vi "analog Handler.vi"(0 "Variable Index":i32, 1 "Action":T2, 5 "End Tid":dbl, 7 "Value":dbl, 9 "Upd freq":T1, 11 "error in (no error)":errorcluster, 12 "Start tid / buf size":dbl, 13 "Initial Data":dbl[](array[numeric])) -> (3 "Indexes":i32[](array[numeric]), 6 "Value out":dbl, 8 "Waveform":waveform(sgl), 10 "Values":dbl[](array[numeric]), 14 "Numb var":i32, 15 "error out":errorcluster)   [LabVIEW 2011]
uses:
  Action Analog Handler.ctl
  Update frequensies.ctl
  Analog Psudo WF.ctl
panel:
  out "Time Stamp":timestamp
  # "OBS, \nBruk Value som oppdaterings frekvens \nunder reg new var."
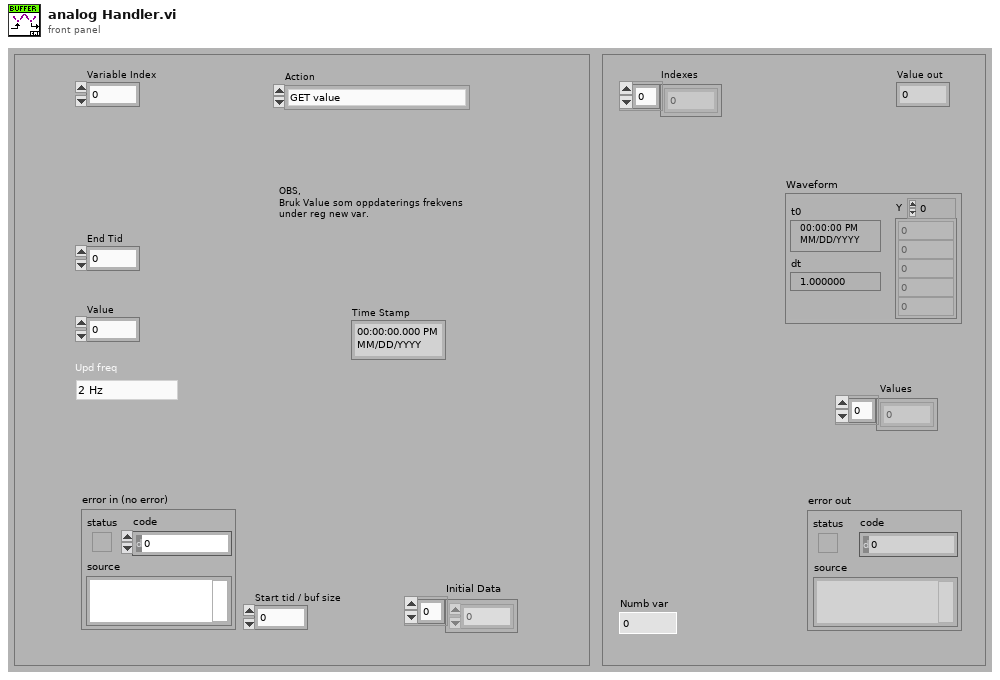
[diagram p1: front panel]
types:
  T1 = typedef "Update frequensies.ctl" = enum16{"2 Hz", "1 Hz", "0.1 Hz"}
  T2 = typedef "Action Analog Handler.ctl" = enum16{"GET value", "GET Single Frequenzy", "GET All Values", "GET Waveform", "Get Numb Var", "SET Value", "START Buffer", "REG Variable", "BUF size(total antal sekund)", "PULS", "Get a Value at time", "Set initial waveform"}
  T3 = typedef "Analog Psudo WF.ctl" = cluster{"\ndata":sgl[], "Index":i32, "Upd freq":T1, "Last index time":dbl, "Rounded":bool}
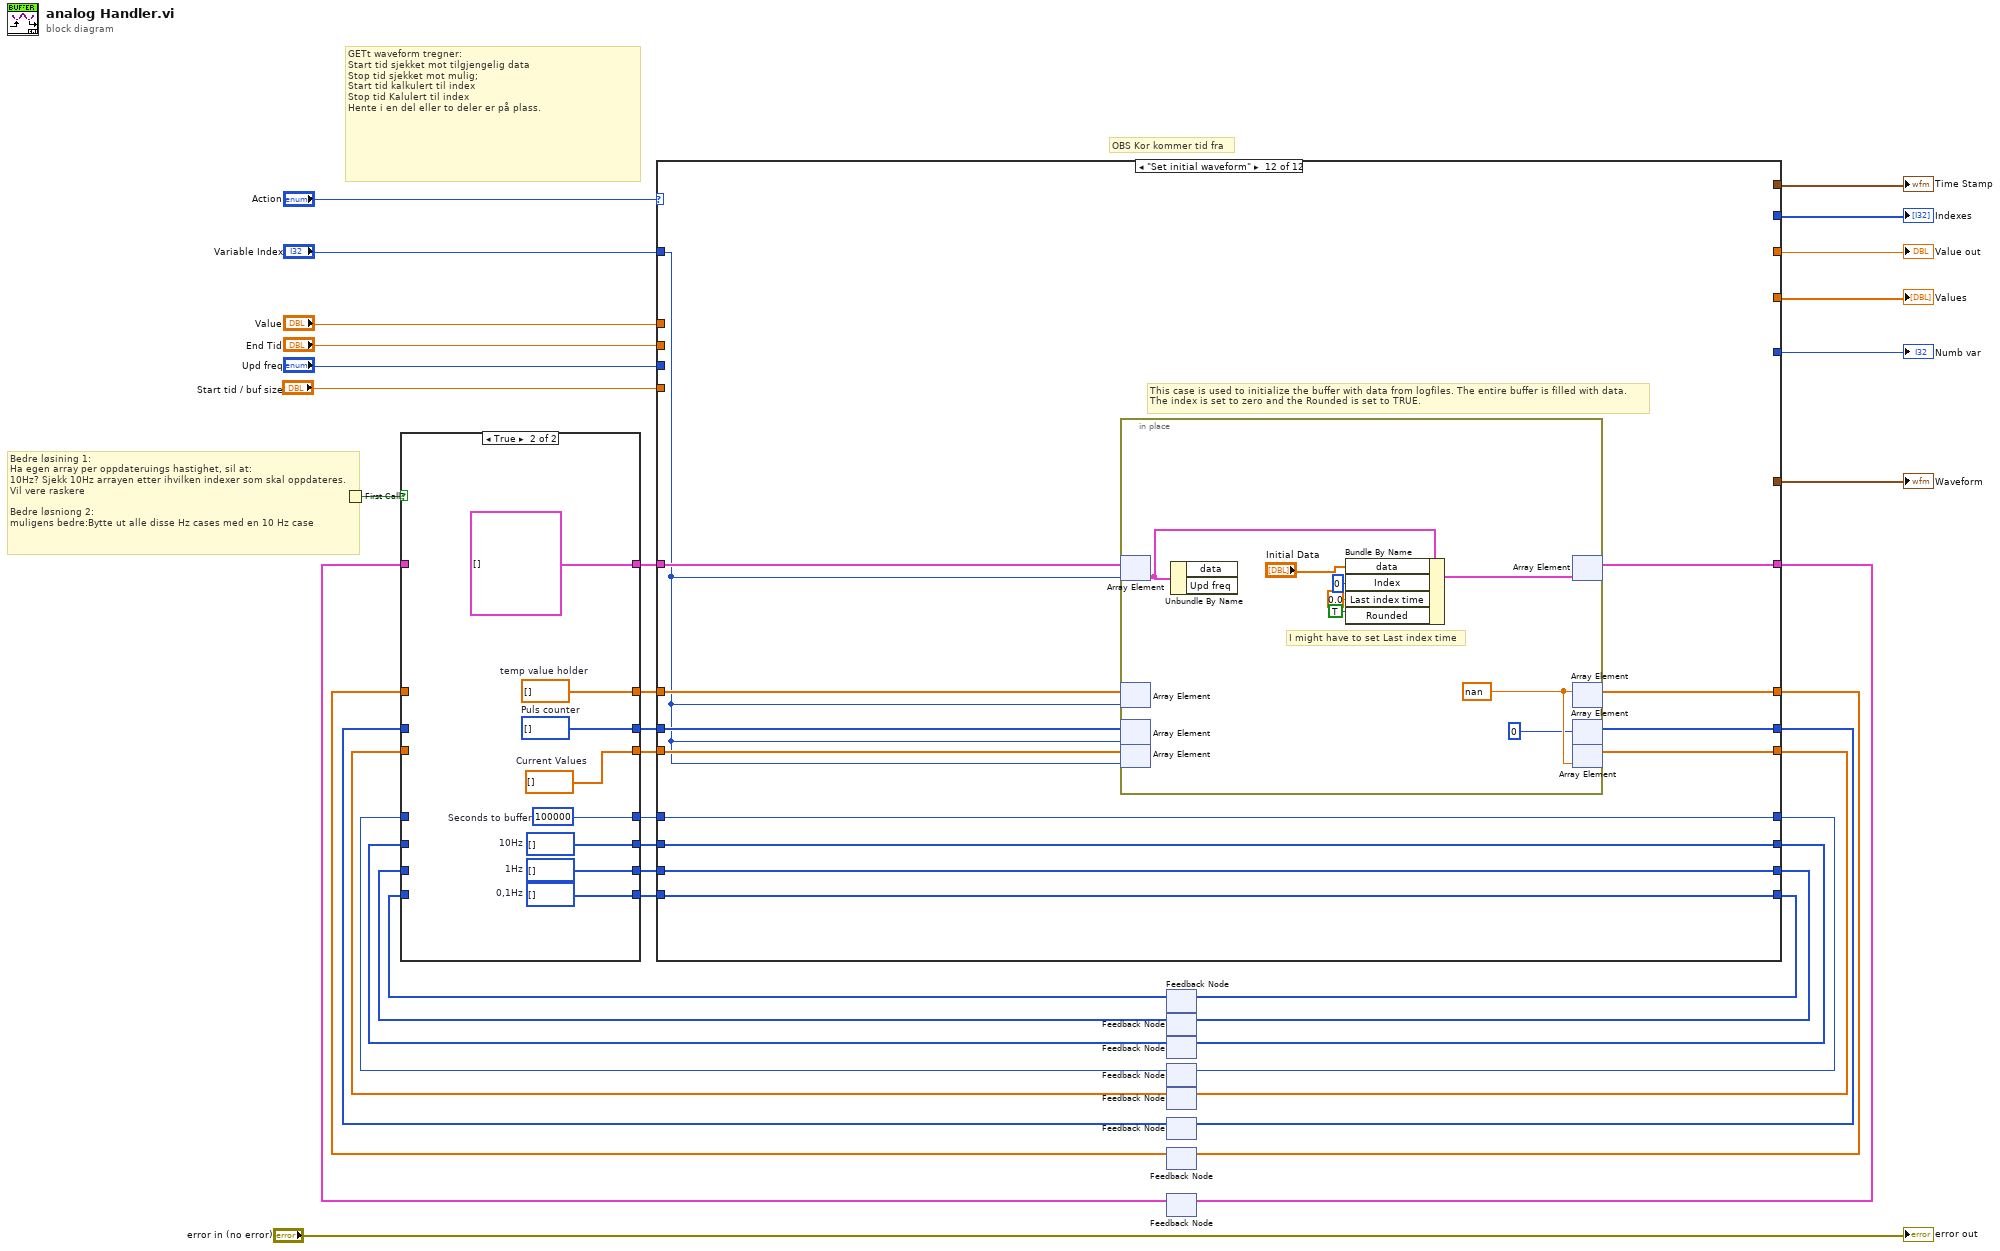
[diagram p0: block diagram]
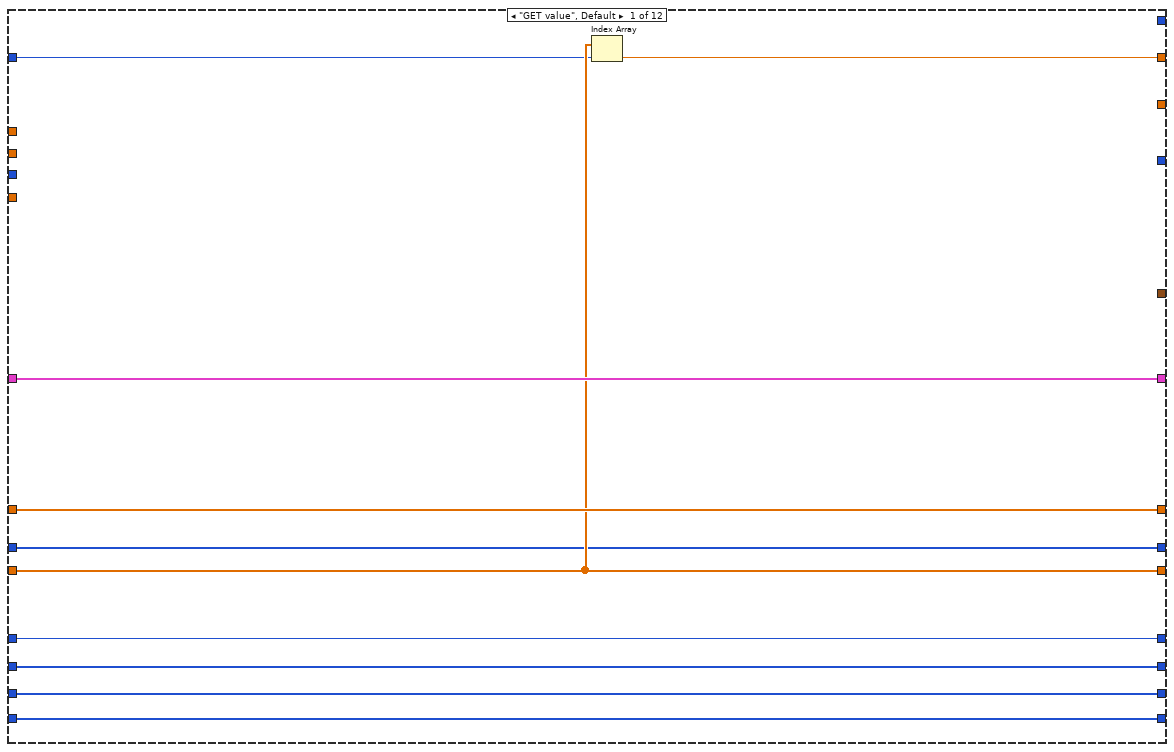
[diagram p3: hidden frame]
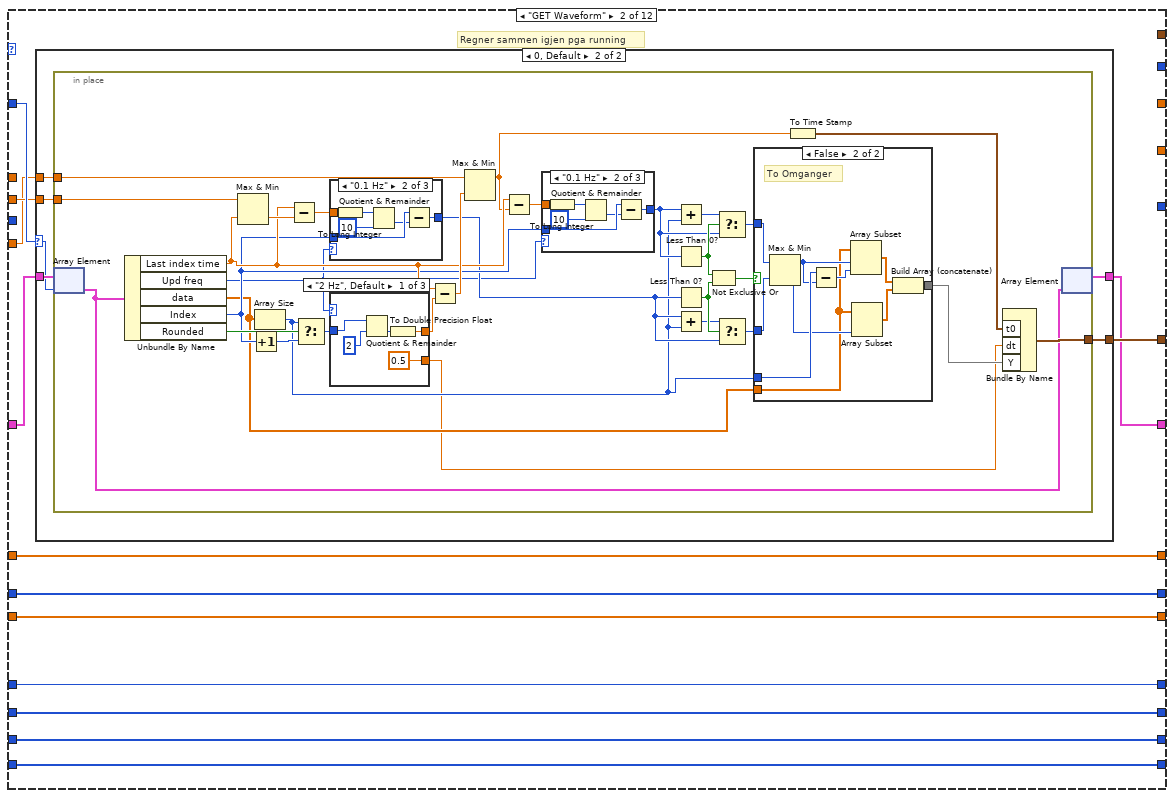
[diagram p4: hidden frame]
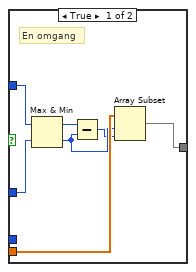
[diagram p6: hidden frame]
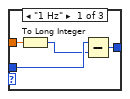
[diagram p7: hidden frame]
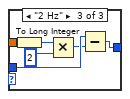
[diagram p8: hidden frame]
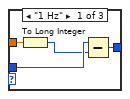
[diagram p9: hidden frame]
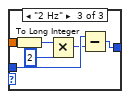
[diagram p10: hidden frame]
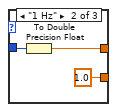
[diagram p11: hidden frame]
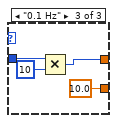
[diagram p12: hidden frame]
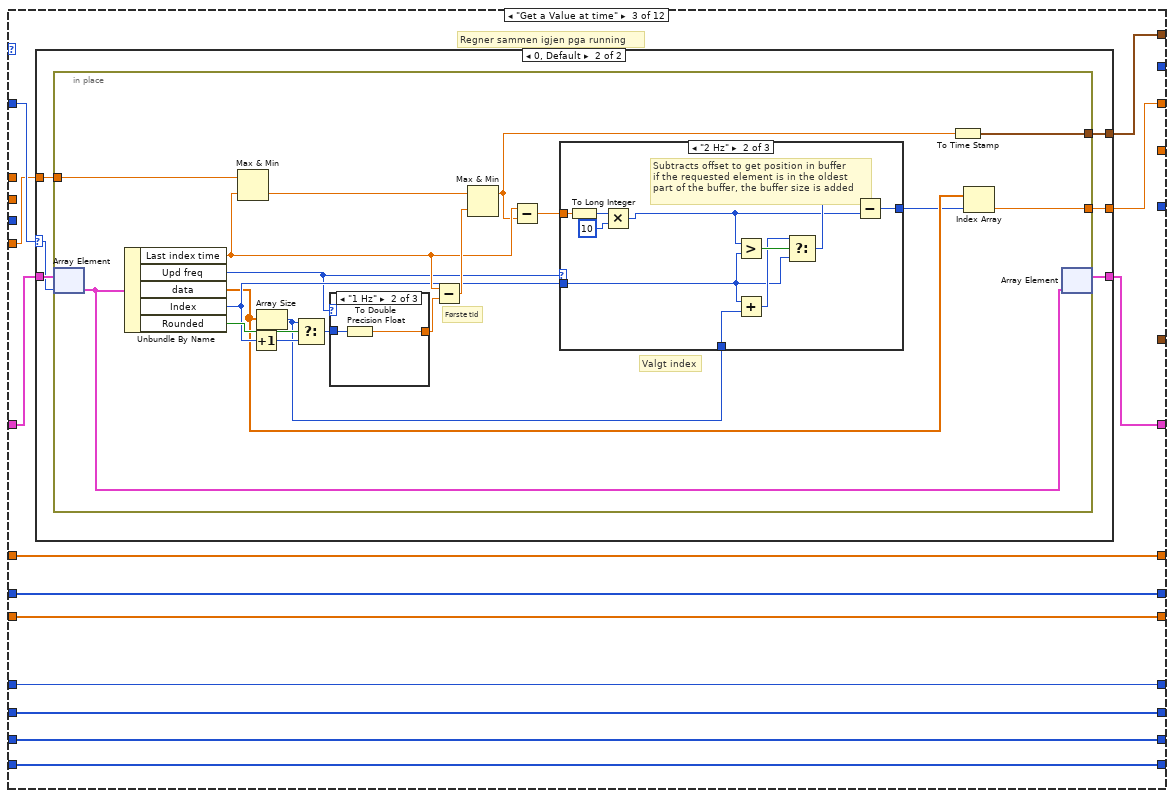
[diagram p13: hidden frame]
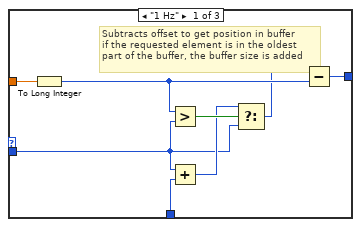
[diagram p15: hidden frame]
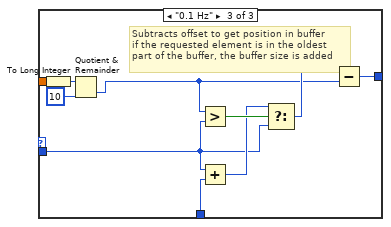
[diagram p16: hidden frame]
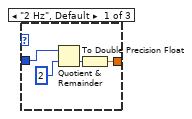
[diagram p17: hidden frame]
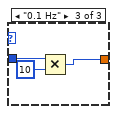
[diagram p18: hidden frame]
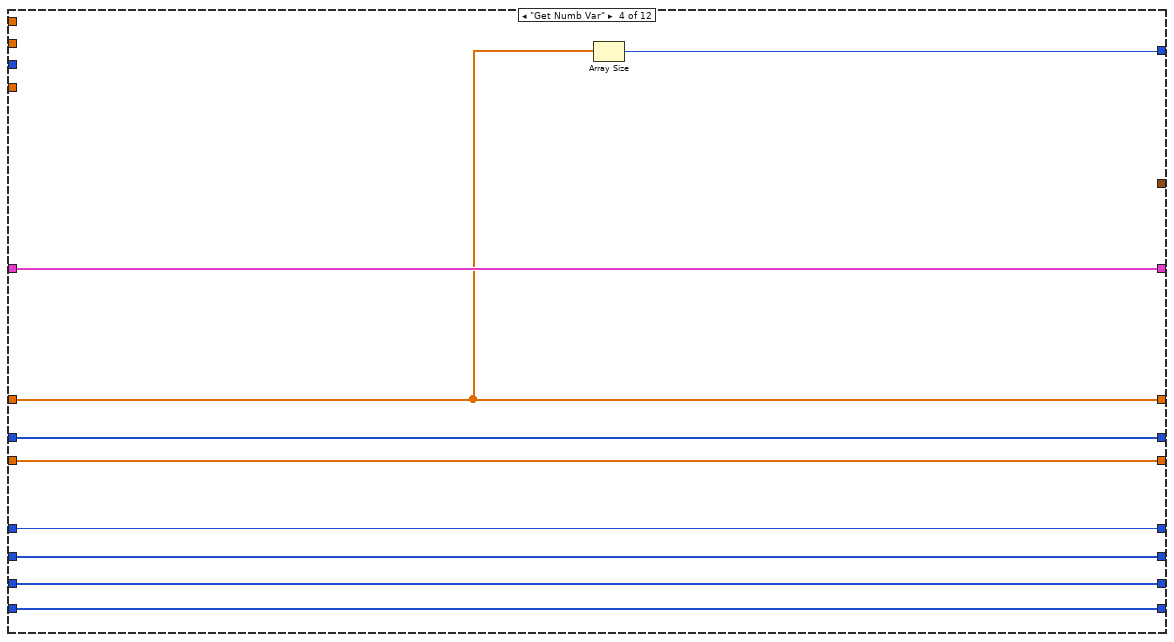
[diagram p19: hidden frame]
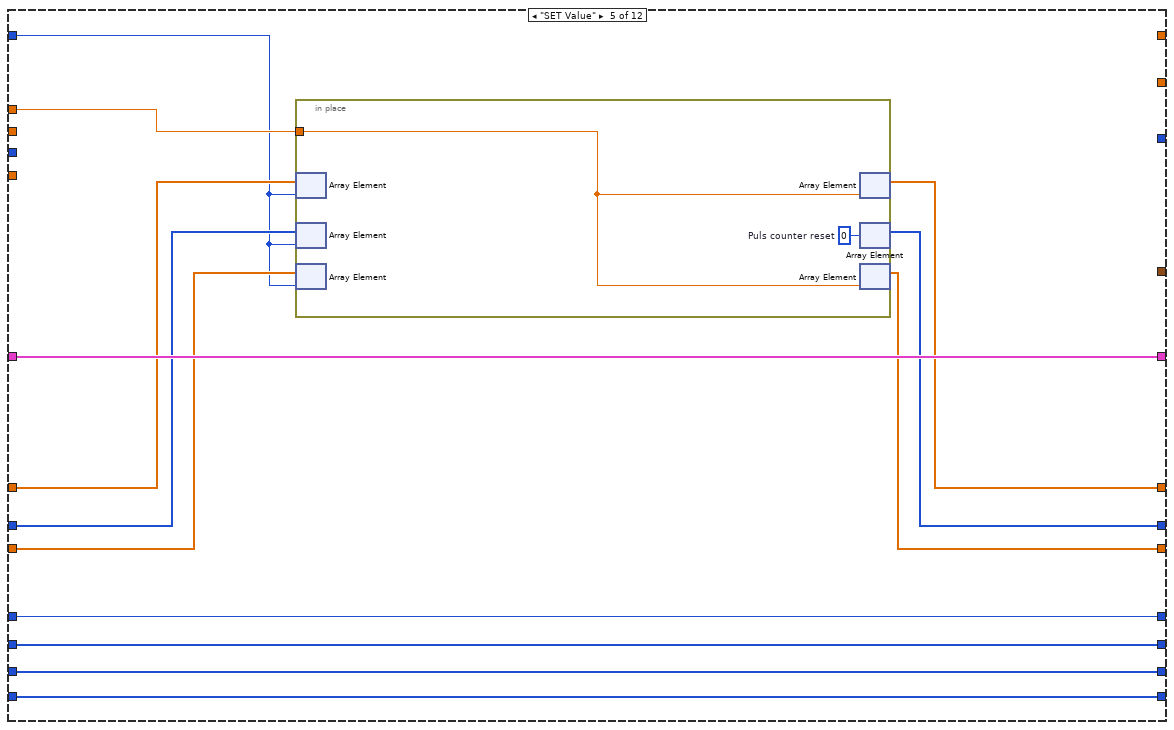
[diagram p20: hidden frame]
diagram:
  # "GETt waveform tregner:\nStart tid sjekket mot tilgjengelig data\nStop tid sjekket mot mulig;\nStart tid kalkulert til index\nStop tid Kalulert til index\nHente i en del eller to deler er på plass."
  # "OBS Kor kommer tid fra"
  # "Bedre løsining 1:\nHa egen array per oppdateruings hastighet, sil at:\n10Hz? Sjekk 10Hz arrayen etter ihvilken indexer som skal oppdateres.\nVil vere raskere\n\nBedre løsniong 2:\nmuligens bedre:Bytte ut alle disse Hz cases med en 10 Hz case"
  n1 = First Call?() -> (First Call?: T/F=w35:bool)
  n2 = feedback #1() -> (w11:i32[])  [unwired: 1 in]
  n3 = feedback #2() -> (w12:i32[])  [unwired: 1 in]
  n4 = feedback #3() -> (w13:i32[])  [unwired: 1 in]
  n5 = feedback #4() -> (w10:i32)  [unwired: 1 in]
  n6 = feedback #5() -> (w27:sgl[])  [unwired: 1 in]
  n7 = feedback #6() -> (w1:u8[])  [unwired: 1 in]
  n8 = feedback #7() -> (w28:sgl[])  [unwired: 1 in]
  n9 = feedback #8() -> (w36:T3[])  [unwired: 1 in]
  n10 = case shown="True" w35 {
    tunnel: w36 -> [w46 _]
    tunnel: [w46 T3[] []] -> w33
    tunnel: [w45 w54] -> w32
    tunnel: [w44 w53] -> w31
    tunnel: w28 -> [w45 _]
    tunnel: w27 -> [w44 _]
    tunnel: [w40 w52] -> w25
    tunnel: [w43 w51] -> w19
    tunnel: [w42 w50] -> w16
    tunnel: [w41 w49] -> w14
    tunnel: w13 -> [w43 _]
    tunnel: w12 -> [w42 _]
    tunnel: w11 -> [w41 _]
    tunnel: w10 -> [w40 _]
    tunnel: [w39 w47] -> w3
    tunnel: w1 -> [w39 _]
    frame False {
    }
    frame True {
      w47 = u8[] []  # Puls counter
      w49 = i32[] []  # 0,1Hz
      w50 = i32[] []  # 1Hz
      w51 = i32[] []  # 10Hz
      w52 = 100000  # Seconds to buffer
      w53 = sgl[] []  # Current Values
      w54 = sgl[] []  # temp value holder
    }
  }
  n11 = case shown="\"Set initial waveform\"" "Action" {
    tunnel: [w64 w69 w181 w259 w272 w283 w300 w359 w386 w417 w489 w512] -> w34
    tunnel: w33 -> [w64 w70 w182 w259 w272 w283 w299 w359 w386 w422 w492 w515]
    tunnel: w32 -> [w63 w77 w188 w252 w270 w282 w297 w360 w388 w399 w491 w514]
    tunnel: w31 -> [w62 w76 w187 w258 w262 w281 w284 w366 w382 w418 w490 w513]
    tunnel: [w63 w77 w188 w252 w269 w282 w298 w360 w388 w416 w488 w511] -> w29
    tunnel: [w62 w76 w187 w258 w260 w281 w296 w367 w382 w415 w487 w510] -> w30
    tunnel: [w59 w67 w180 w257 w271 w277 w295 w365 w387 w397 w493 w516] -> w26
    tunnel: w25 -> [w59 w67 w180 w257 w271 _ w295 w365 w387 w397 w493 w516]
    tunnel: "Variable Index" -> [w60 w71 w183 _ w261 _ _ _ _ w398 w482 w505]
    tunnel: "Value" -> [_ _ _ _ w268 _ _ _ _ _ _ _]
    tunnel: [w61 _ w178 _ _ _ _ _ _ _ _ _] -> w22
    tunnel: [_ _ _ _ _ _ w289 w357 w382 _ _ _] -> w21
    tunnel: [_ _ _ w256 _ _ w290 w358 _ _ _ _] -> w20
    tunnel: w19 -> [w58 w75 w186 w255 w267 w280 w292 w362 w385 w411 w486 w509]
    tunnel: [w58 w75 w186 w255 w267 w280 w292 w362 w385 w405 w486 w509] -> w18
    tunnel: [w57 w74 w185 w254 w266 w279 w294 w364 w384 w402 w485 w508] -> w17
    tunnel: w16 -> [w57 w74 w185 w254 w266 w279 w294 w364 w384 w410 w485 w508]
    tunnel: [w56 w73 w184 w253 w265 w278 w293 w363 w383 w400 w484 w507] -> w15
    tunnel: w14 -> [w56 w73 w184 w253 w265 w278 w293 w363 w383 w409 w484 w507]
    tunnel: [_ w72 _ _ _ _ _ _ _ _ _ _] -> w8
    tunnel: "Upd freq" -> [_ _ _ _ _ _ w291 w361 _ w394 _ _]
    tunnel: [_ _ _ _ _ _ w288 w356 w381 _ _ _] -> w7
    tunnel: "End Tid" -> [_ w68 _ _ _ _ _ _ _ _ _ _]
    tunnel: [_ _ w179 _ _ _ _ _ _ _ _ _] -> w5
    tunnel: "Start tid / buf size" -> [_ w66 w177 _ _ w276 w287 _ _ _ _ _]
    tunnel: w3 -> [w55 w65 w176 w251 w264 w275 w286 w355 w380 w392 w483 w506]
    tunnel: [w55 w65 w176 w251 w263 w275 w285 w355 w380 w391 w481 w504] -> w2
    frame "GET value", Default {
      n12 = Index Array(array=w62, index=w60) -> (element=w61:sgl)
    }
    frame "GET Waveform" {
      # "Regner sammen igjen pga running"
      n13 = case shown="0, Default" w71 {
        selector: w71 -> [_ w81]
        tunnel: w70 -> [w78 w82]
        tunnel: w66 -> [_ w84]
        tunnel: [_ w83] -> w72
        tunnel: [w78 w80] -> w69
        tunnel: w68 -> [_ w79]
        frame ..-1 {
        }
        frame 0, Default {
          n14 = in-place {
            in-place-border: w84 -> [w112]
            in-place-border: [w114] -> w83
            in-place-border: w79 -> [w111]
            n15 = in-place-array #9(w82, w81) -> (w113:T3)
            n16 = Unbundle By Name(w113) -> ("Last index time"=w103:dbl, "Upd freq"=w85:T1, "data"=w91:sgl[], "Index"=w101:i32, "Rounded"=w110:bool)
            n17 = Max & Min(x=w111, y=w103) -> (min(x,y)=w105:dbl)  [unwired: 1 out]
            n18 = Increment(x=w101) -> (x+1=w109:i32)
            n19 = Array Size(array=w91) -> (size(s)=w89:i32)
            n20 = Subtract(x=w103, y=w105) -> (x-y=w104:dbl)
            n21 = Select(t=w89, s=w110, f=w109) -> (s? t:f=w108:i32)
            n22 = case shown="\"0.1 Hz\"" w85 {
              tunnel: w101 -> [w150 w156 w162]
              tunnel: w104 -> [w151 w157 w163]
              tunnel: [w148 w154 w160] -> w98
              frame "1 Hz" {
                n23 = To Long Integer(number=w151) -> (32bit integer=w149:i32)
                n24 = Subtract(x=w150, y=w149) -> (x-y=w148:i32)
              }
              frame "0.1 Hz" {
                n25 = To Long Integer(number=w157) -> (32bit integer=w155:i32)
                n26 = Quotient & Remainder(x=w155, y=10) -> (floor(x/y)=w153:i32)  [unwired: 1 out]
                n27 = Subtract(x=w156, y=w153) -> (x-y=w154:i32)
              }
              frame "2 Hz" {
                n28 = To Long Integer(number=w163) -> (32bit integer=w161:i32)
                n29 = Multiply(x=w161, y=2) -> (x*y=w159:i32)
                n30 = Subtract(x=w162, y=w159) -> (x-y=w160:i32)
              }
            }
            n31 = case shown="\"2 Hz\", Default" w85 {
              tunnel: w108 -> [w168 w171 w175]
              tunnel: [w167 w170 w173] -> w107
              tunnel: [0.5 ("dt") 1.0 ("dt") 10.0 ("dt")] -> w88
              frame "2 Hz", Default {
                n32 = Quotient & Remainder(x=w168, y=2 ("x")) -> (floor(x/y)=w166:i32)  [unwired: 1 out]
                n33 = To Double Precision Float(number=w166) -> (double precision float=w167:dbl)
              }
              frame "1 Hz" {
                n34 = To Double Precision Float(number=w171) -> (double precision float=w170:dbl)
              }
              frame "0.1 Hz" {
                n35 = Multiply(x=w175, y=10) -> (x*y=w173:i32)
              }
            }
            n36 = Subtract(x=w103, y=w107) -> (x-y=w106:dbl)
            n37 = Max & Min(x=w112, y=w106) -> (max(x,y)=w87:dbl)  [unwired: 1 out]
            n38 = Subtract(x=w103, y=w87) -> (x-y=w102:dbl)
            n39 = case shown="\"0.1 Hz\"" w85 {
              tunnel: w101 -> [w134 w140 w146]
              tunnel: w102 -> [w135 w141 w147]
              tunnel: [w132 w138 w144] -> w95
              frame "1 Hz" {
                n40 = To Long Integer(number=w135) -> (32bit integer=w133:i32)
                n41 = Subtract(x=w134, y=w133) -> (x-y=w132:i32)
              }
              frame "0.1 Hz" {
                n42 = To Long Integer(number=w141) -> (32bit integer=w139:i32)
                n43 = Quotient & Remainder(x=w139, y=10) -> (floor(x/y)=w137:i32)  [unwired: 1 out]
                n44 = Subtract(x=w140, y=w137) -> (x-y=w138:i32)
              }
              frame "2 Hz" {
                n45 = To Long Integer(number=w147) -> (32bit integer=w145:i32)
                n46 = Multiply(x=w145, y=2) -> (x*y=w143:i32)
                n47 = Subtract(x=w146, y=w143) -> (x-y=w144:i32)
              }
            }
            n48 = Add(x=w95, y=w89) -> (x+y=w96:i32)
            n49 = Less Than 0?(x=w95) -> (x < 0?=w100:bool)
            n50 = Less Than 0?(x=w98) -> (x < 0?=w99:bool)
            n51 = Add(x=w98, y=w89) -> (x+y=w97:i32)
            n52 = Not Exclusive Or(1:w99, 2:w100) -> (0:w94:bool)
            n53 = Select(t=w96, s=w100, f=w95) -> (s? t:f=w93:i32)
            n54 = Select(t=w97, s=w99, f=w98) -> (s? t:f=w92:i32)
            n55 = case shown="False" w94 {
              tunnel: w93 -> [w121 w131]
              tunnel: w92 -> [w120 w130]
              tunnel: w91 -> [w118 w125]
              tunnel: [w115 w122] -> w90
              tunnel: w89 -> [_ w129]
              frame True {
                # "En omgang"
                n56 = Max & Min(x=w121, y=w120) -> (max(x,y)=w119:i32, min(x,y)=w117:i32)
                n57 = Subtract(x=w119, y=w117) -> (x-y=w116:i32)
                n58 = Array Subset(array=w118, index=w117, length=w116) -> (w115:sgl[])
              }
              frame False {
                # "To Omganger"
                n59 = Max & Min(x=w131, y=w130) -> (max(x,y)=w128:i32, min(x,y)=w126:i32)
                n60 = Subtract(x=w129, y=w128) -> (x-y=w127:i32)
                n61 = Array Subset(array=w125, index=w128, length=w127) -> (w124:sgl[])
                n62 = Array Subset(array=w125, length=w126) -> (w123:sgl[])  [unwired: 1 in]
                n63 = Build Array (concatenate)(w124, w123) -> (w122:sgl[])
              }
            }
            n64 = To Time Stamp(1:w87) -> (0:w86:timestamp)
            n65 = Bundle By Name("t0"=w86, "dt"=w88, "Y"=w90) -> (w114:waveform(sgl))  [unwired: 1 in]
            n66 = in-place-array #9(w113) -> (w80:T3[])  [unwired: 1 out]
          }
        }
      }
    }
    frame "Get a Value at time" {
      # "Regner sammen igjen pga running"
      n67 = case shown="0, Default" w183 {
        selector: w183 -> [_ w193]
        tunnel: w182 -> [w189 w194]
        tunnel: w177 -> [_ w195]
        tunnel: [w189 w192] -> w181
        tunnel: [_ w191] -> w179
        tunnel: [_ w190] -> w178
        frame ..-1 {
        }
        frame 0, Default {
          n68 = in-place {
            in-place-border: w195 -> [w212]
            in-place-border: [w198] -> w191
            in-place-border: [w197] -> w190
            # "Valgt index"
            # "Første tid"
            n69 = in-place-array #10(w194, w193) -> (w213:T3)
            n70 = Unbundle By Name(w213) -> ("Last index time"=w206:dbl, "Upd freq"=w202:T1, "data"=w200:sgl[], "Index"=w204:i32, "Rounded"=w211:bool)
            n71 = Max & Min(x=w212, y=w206) -> (min(x,y)=w201:dbl)  [unwired: 1 out]
            n72 = Increment(x=w204) -> (x+1=w210:i32)
            n73 = Array Size(array=w200) -> (size(s)=w196:i32)
            n74 = Select(t=w196, s=w211, f=w210) -> (s? t:f=w209:i32)
            n75 = case shown="\"1 Hz\"" w202 {
              tunnel: w209 -> [w245 w247 w250]
              tunnel: [w244 w246 w248] -> w208
              frame "2 Hz", Default {
                n76 = Quotient & Remainder(x=w245, y=2 ("x")) -> (floor(x/y)=w243:i32)  [unwired: 1 out]
                n77 = To Double Precision Float(number=w243) -> (double precision float=w244:dbl)
              }
              frame "1 Hz" {
                n78 = To Double Precision Float(number=w247) -> (double precision float=w246:dbl)
              }
              frame "0.1 Hz" {
                n79 = Multiply(x=w250, y=10) -> (x*y=w248:i32)
              }
            }
            n80 = Subtract(x=w206, y=w208) -> (x-y=w207:dbl)
            n81 = Max & Min(x=w201, y=w207) -> (max(x,y)=w203:dbl)  [unwired: 1 out]
            n82 = Subtract(x=w206, y=w203) -> (x-y=w205:dbl)
            n83 = case shown="\"2 Hz\"" w202 {
              tunnel: w204 -> [w216 w228 w238]
              tunnel: w205 -> [w221 w223 w233]
              tunnel: [w220 w231 w241] -> w199
              tunnel: w196 -> [w214 w226 w236]
              frame "1 Hz" {
                # "Subtracts offset to get position in buffer\nif the requested element is in the oldest\npart of the buffer, the buffer size is added"
                n84 = To Long Integer(number=w221) -> (32bit integer=w219:i32)
                n85 = Greater?(x=w219, y=w216) -> (0:w218:bool)
                n86 = Add(x=w216, y=w214) -> (x+y=w217:i32)
                n87 = Select(t=w217, s=w218, f=w216) -> (s? t:f=w215:i32)
                n88 = Subtract(x=w215, y=w219) -> (x-y=w220:i32)
              }
              frame "2 Hz" {
                # "Subtracts offset to get position in buffer\nif the requested element is in the oldest\npart of the buffer, the buffer size is added"
                n89 = To Long Integer(number=w223) -> (32bit integer=w225:i32)
                n90 = Multiply(x=w225, y=10) -> (x*y=w222:i32)
                n91 = Greater?(x=w222, y=w228) -> (0:w230:bool)
                n92 = Add(x=w228, y=w226) -> (x+y=w229:i32)
                n93 = Select(t=w229, s=w230, f=w228) -> (s? t:f=w227:i32)
                n94 = Subtract(x=w227, y=w222) -> (x-y=w231:i32)
              }
              frame "0.1 Hz" {
                # "Subtracts offset to get position in buffer\nif the requested element is in the oldest\npart of the buffer, the buffer size is added"
                n95 = To Long Integer(number=w233) -> (32bit integer=w235:i32)
                n96 = Quotient & Remainder(x=w235, y=10) -> (floor(x/y)=w232:i32)  [unwired: 1 out]
                n97 = Greater?(x=w232, y=w238) -> (0:w240:bool)
                n98 = Add(x=w238, y=w236) -> (x+y=w239:i32)
                n99 = Select(t=w239, s=w240, f=w238) -> (s? t:f=w237:i32)
                n100 = Subtract(x=w237, y=w232) -> (x-y=w241:i32)
              }
            }
            n101 = To Time Stamp(1:w203) -> (0:w198:timestamp)
            n102 = Index Array(array=w200, index=w199) -> (element=w197:sgl)
            n103 = in-place-array #10(w213) -> (w192:T3[])  [unwired: 1 out]
          }
        }
      }
    }
    frame "Get Numb Var" {
      n104 = Array Size(array=w252) -> (size(s)=w256:i32)
    }
    frame "SET Value" {
      n105 = in-place {
        in-place-border: w268 -> [w273]
        w274 = u8 0  # Puls counter reset
        n106 = in-place-array #11(w270, w261) -> ()  [unwired: 1 out]
        n107 = in-place-array #12(w264, w261) -> ()  [unwired: 1 out]
        n108 = in-place-array #13(w262, w261) -> ()  [unwired: 1 out]
        n109 = in-place-array #11(w273) -> (w269:sgl[])  [unwired: 1 out]
        n110 = in-place-array #12(w274) -> (w263:u8[])  [unwired: 1 out]
        n111 = in-place-array #13(w273) -> (w260:sgl[])  [unwired: 1 out]
      }
    }
    frame "BUF size(total antal sekund)" {
      n112 = To Long Integer(number=w276) -> (32bit integer=w277:i32)
    }
    frame "PULS" {
      n113 = case shown="\"1 Hz\"" w291 {
        tunnel: w292 -> [_ w303 _]
        tunnel: w294 -> [_ _ w304]
        tunnel: w293 -> [w302 _ _]
        tunnel: [w302 w303 w304] -> w288
        frame "0.1 Hz" {
        }
        frame "2 Hz" {
        }
        frame "1 Hz" {
        }
      }
      n114 = Empty Array?(array=w288) -> (empty?=w301:bool)
      n115 = case shown="False" w301 {
        tunnel: [w311 w354] -> w300
        tunnel: w299 -> [w313 w354]
        tunnel: [w310 w353] -> w298
        tunnel: w297 -> [w314 w353]
        tunnel: [w309 w352] -> w296
        tunnel: w284 -> [w315 w352]
        tunnel: w288 -> [w312 _]
        tunnel: w287 -> [w308 _]
        tunnel: [w307 _] -> w289
        tunnel: w286 -> [w306 w351]
        tunnel: [w305 w351] -> w285
        frame False {
          n116 = for {
            tunnel: w312 -> [w317] mode=indexing
            shift-right: [w321] -> w311
            shift-left: w313 -> [w322]
            shift-right: [w323] -> w310
            shift-left: w314 -> [w324]
            shift-right: [w325] -> w309
            shift-left: w315 -> [w326]
            tunnel: w308 -> [w320]
            tunnel: [w319] -> w307 mode=indexing
            shift-right: [w316] -> w305
            shift-left: w306 -> [w318]
            n117 = in-place {
              in-place-border: w320 -> [w334]
              in-place-border: [w332] -> w319
              # "Sets values to NaN if data has not been updated since the 5\nlast pulses"
              n118 = in-place-array #14(w322, w317) -> (w336:T3)
              n119 = in-place-array #15(w324, w317) -> (w332:sgl)
              n120 = in-place-array #16(w318, w317) -> (w330:u8)
              n121 = in-place-array #17(w326, w317) -> ()  [unwired: 1 out]
              n122 = in-place {
                in-place-border: w332 -> [w342]
                in-place-border: w334 -> [w341]
                # "Antall skal ikke endre seg"
                n123 = in-place-cluster #18(w336) -> ("data"=w345:sgl[], "Index"=w343:i32, "Rounded"=w340:bool)  [unwired: 1 out]
                n124 = in-place {
                  in-place-border: w342 -> [w350]
                  n125 = in-place-array #19(w345, w343) -> ()  [unwired: 1 out]
                  n126 = in-place-array #19(w350) -> (w344:sgl[])  [unwired: 1 out]
                }
                n127 = Array Size(array=w345) -> (size(s)=w349:i32)
                n128 = Increment(x=w343) -> (x+1=w348:i32)
                n129 = Greater Or Equal?(x=w348, y=w349) -> (x >= y?=w339:bool)
                n130 = Select(t=0, s=w339, f=w348) -> (s? t:f=w346:i32)
                n131 = Or(x=w339, y=w340) -> (x .or. y?=w338:bool)
                n132 = in-place-cluster #18("Last index time"=w341, "data"=w344, "Index"=w346, "Rounded"=w338) -> (w335:T3)
              }
              n133 = Greater Or Equal?(x=w330, y=u8 5) -> (x >= y?=w331:bool)
              n134 = Select(t=sgl nan ("element"), s=w331, f=w332) -> (s? t:f=w333:sgl)
              n135 = Increment(x=w330) -> (x+1=w329:u8)
              n136 = Select(t=w330, s=w331, f=w329) -> (s? t:f=w328:u8)
              n137 = in-place-array #14(w335) -> (w321:T3[])  [unwired: 1 out]
              n138 = in-place-array #15(w333) -> (w323:sgl[])  [unwired: 1 out]
              n139 = in-place-array #16(w328) -> (w316:u8[])  [unwired: 1 out]
              n140 = in-place-array #17(w332) -> (w325:sgl[])  [unwired: 1 out]
            }
          }
        }
        frame True {
          # "Ingen 10 Hzere"
        }
      }
      n141 = Array Size(array=w289) -> (size(s)=w290:i32)
    }
    frame "GET Single Frequenzy" {
      n142 = case shown="\"0.1 Hz\"" w361 {
        tunnel: w362 -> [_ w370 _]
        tunnel: w364 -> [_ _ w371]
        tunnel: w363 -> [w369 _ _]
        tunnel: [w369 w370 w371] -> w356
        frame "0.1 Hz" {
        }
        frame "2 Hz" {
        }
        frame "1 Hz" {
        }
      }
      n143 = Empty Array?(array=w356) -> (empty?=w368:bool)
      n144 = case shown="False" w368 {
        tunnel: [w374 w379] -> w367
        tunnel: w366 -> [w375 w379]
        tunnel: w356 -> [w373 _]
        tunnel: [w372 _] -> w357
        frame False {
          n145 = for {
            shift-right: [w377] -> w374
            shift-left: w375 -> [w377]
            tunnel: w373 -> [w378] mode=indexing
            tunnel: [w376] -> w372 mode=indexing
            n146 = Index Array(array=w377, index=w378) -> (element=w376:sgl)
          }
        }
        frame True {
        }
      }
      n147 = Array Size(array=w357) -> (size(s)=w358:i32)
    }
    frame "GET All Values" {
      n148 = for {
        tunnel: w382 -> [_] mode=indexing
        tunnel: [w389] -> w381 mode=indexing
        i -> [w389]
      }
    }
    frame "REG Variable" {
      # "Fjerner den nye, om den ligger i en av listene"
      n149 = To Long Integer(number=w398) -> (32bit integer=w390:i32)
      n150 = Increment(x=w390) -> (x+1=w413:i32)
      n151 = Search 1D Array(1D array=w409, element=w390) -> (index of element=w408:i32)  [unwired: 1 in]
      n152 = Array Size(array=w399) -> (size(s)=w414:i32)
      n153 = Subtract(x=w413, y=w414) -> (x-y=w412:i32)
      n154 = Delete From Array(array=w409, index=w408) -> (array with subset deleted=w401:i32[])  [unwired: 1 in, 1 out]
      n155 = Search 1D Array(1D array=w410, element=w390) -> (index of element=w406:i32)  [unwired: 1 in]
      n156 = case shown="\"0.1 Hz\"" w394 {
        selector: w394 -> [w423 w427 w431]
        tunnel: w397 -> [w426 w430 w432]
        tunnel: [w424 w428 w432] -> w396
        tunnel: [w423 w427 w431] -> w395
        frame "2 Hz" {
          n157 = Multiply(x=w426, y=2) -> (x*y=w424:i32)
        }
        frame "0.1 Hz" {
          n158 = Quotient & Remainder(x=w430, y=10) -> (floor(x/y)=w428:i32)  [unwired: 1 out]
        }
        frame "1 Hz" {
        }
      }
      n159 = Delete From Array(array=w410, index=w406) -> (array with subset deleted=w403:i32[])  [unwired: 1 in, 1 out]
      n160 = case shown="1, Default" w412 {
        selector: w412 -> [_ w452]
        tunnel: w422 -> [w451 w472]
        tunnel: [w451 w471] -> w421
        tunnel: [w450 w457] -> w420
        tunnel: w399 -> [w450 w469]
        tunnel: [w449 w470] -> w419
        tunnel: w418 -> [w449 w468]
        tunnel: w396 -> [_ w460]
        tunnel: w395 -> [_ w459]
        tunnel: [w448 w455] -> w393
        tunnel: w392 -> [w448 w456]
        frame 0 {
        }
        frame 1, Default {
          w458 = sgl nan
          (unwired) sgl 0.0
          (unwired) sgl 0.0
          # "20110707"
          n161 = Initialize Array(sgl nan, w460) -> (w462:sgl[])
          n162 = Bundle By Name(cluster=T3 {"\ndata"=[], "Index"=0, "Upd freq"=enum."2 Hz", "Last index time"=0.0, "Rounded"=FALSE} ("Psudu Wf"), "data"=w462, "Upd freq"=w459) -> (w461:T3)
          n163 = Initialize Array(w458, w452) -> (w465:sgl[])
          n164 = Initialize Array(w461, w452) -> (w467:T3[])
          n165 = Initialize Array(w458, w452) -> (w466:sgl[])
          n166 = Initialize Array(u8 0 ("element"), w452) -> (w454:u8[])
          n167 = Build Array (concatenate)(w472, w467) -> (w471:T3[])
          n168 = Build Array (concatenate)(w469, w466) -> (w457:sgl[])
          n169 = Build Array (concatenate)(w456, w454) -> (w455:u8[])
          n170 = Build Array (concatenate)(w468, w465) -> (w470:sgl[])
        }
      }
      n171 = Search 1D Array(1D array=w411, element=w390) -> (index of element=w407:i32)  [unwired: 1 in]
      n172 = Delete From Array(array=w411, index=w407) -> (array with subset deleted=w404:i32[])  [unwired: 1 in, 1 out]
      n173 = case shown="\"2 Hz\"" w394 {
        tunnel: [w437 w439 w447] -> w405
        tunnel: w404 -> [w437 w442 w447]
        tunnel: w403 -> [w436 w441 w446]
        tunnel: [w436 w441 w444] -> w402
        tunnel: w401 -> [w435 w440 w445]
        tunnel: [w434 w440 w445] -> w400
        tunnel: w390 -> [w433 w438 w443]
        frame "0.1 Hz" {
          n174 = Build Array (concatenate)(w435, w433) -> (w434:i32[])
        }
        frame "2 Hz" {
          n175 = Build Array (concatenate)(w442, w438) -> (w439:i32[])
        }
        frame "1 Hz" {
          n176 = Build Array (concatenate)(w446, w443) -> (w444:i32[])
        }
      }
      n177 = in-place {
        in-place-border: w396 -> [w475]
        in-place-border: w395 -> [w474]
        w480 = nan ("element")
        n178 = in-place-array #20(w421, w390) -> ()  [unwired: 1 out]
        n179 = in-place-array #21(w420, w390) -> ()  [unwired: 1 out]
        n180 = in-place-array #22(w393, w390) -> ()  [unwired: 1 out]
        n181 = in-place-array #23(w419, w390) -> ()  [unwired: 1 out]
        n182 = Initialize Array(sgl nan, w475) -> (w477:sgl[])
        n183 = Bundle By Name(cluster=T3 {"\ndata"=[], "Index"=0, "Upd freq"=enum."2 Hz", "Last index time"=0.0, "Rounded"=FALSE} ("Psudu Wf"), "data"=w477, "Upd freq"=w474) -> (w476:T3)
        n184 = in-place-array #20(w476) -> (w417:T3[])  [unwired: 1 out]
        n185 = in-place-array #21(w480) -> (w416:sgl[])  [unwired: 1 out]
        n186 = in-place-array #22(u8 0 ("element")) -> (w391:u8[])  [unwired: 1 out]
        n187 = in-place-array #23(w480) -> (w415:sgl[])  [unwired: 1 out]
      }
    }
    frame "START Buffer" {
      n188 = in-place {
        w503 = sgl nan ("element")
        n189 = in-place-array #24(w492, w482) -> (w499:T3)
        n190 = in-place-array #25(w491, w482) -> ()  [unwired: 1 out]
        n191 = in-place-array #26(w483, w482) -> ()  [unwired: 1 out]
        n192 = in-place-array #27(w490, w482) -> ()  [unwired: 1 out]
        n193 = Unbundle By Name(w499) -> ("data"=w498:sgl[], "Upd freq"=w494:T1)
        n194 = Array Size(array=w498) -> (size(s)=w497:i32)
        n195 = Initialize Array(sgl nan, w497) -> (w500:sgl[])
        n196 = Bundle By Name(cluster=T3 {"\ndata"=[], "Index"=0, "Upd freq"=enum."2 Hz", "Last index time"=0.0, "Rounded"=FALSE} ("Psudu Wf"), "data"=w500, "Upd freq"=w494) -> (w496:T3)
        n197 = in-place-array #24(w496) -> (w489:T3[])  [unwired: 1 out]
        n198 = in-place-array #25(w503) -> (w488:sgl[])  [unwired: 1 out]
        n199 = in-place-array #26(u8 0 ("element")) -> (w481:u8[])  [unwired: 1 out]
        n200 = in-place-array #27(w503) -> (w487:sgl[])  [unwired: 1 out]
      }
    }
    frame "Set initial waveform" {
      # "This case is used to initialize the buffer with data from logfiles. The entire buffer is filled with data.\nThe index is set to zero and the Rounded is set to TRUE."
      n201 = in-place {
        w524 = sgl nan ("element")
        # "I might have to set Last index time"
        n202 = in-place-array #28(w515, w505) -> (w519:T3)
        n203 = in-place-array #29(w514, w505) -> ()  [unwired: 1 out]
        n204 = in-place-array #30(w506, w505) -> ()  [unwired: 1 out]
        n205 = in-place-array #31(w513, w505) -> ()  [unwired: 1 out]
        n206 = Unbundle By Name(w519) -> ()  [unwired: 2 out]
        n207 = Bundle By Name(cluster=w519, "data"="Initial Data", "Index"=0, "Last index time"=0.0, "Rounded"=TRUE) -> (w523:T3)
        n208 = in-place-array #28(w523) -> (w512:T3[])  [unwired: 1 out]
        n209 = in-place-array #29(w524) -> (w511:sgl[])  [unwired: 1 out]
        n210 = in-place-array #30(u8 0 ("element")) -> (w504:u8[])  [unwired: 1 out]
        n211 = in-place-array #31(w524) -> (w510:sgl[])  [unwired: 1 out]
      }
    }
  }
  "Values" <- w21
  "Value out" <- w22
  "Numb var" <- w20
  "Waveform" <- w8
  "Indexes" <- w7
  "Time Stamp" <- w5
  n212 = feedback-in #1(w15) -> ()
  n213 = feedback-in #2(w17) -> ()
  n214 = feedback-in #3(w18) -> ()
  n215 = feedback-in #4(w26) -> ()
  n216 = feedback-in #5(w30) -> ()
  n217 = feedback-in #6(w2) -> ()
  n218 = feedback-in #7(w29) -> ()
  n219 = feedback-in #8(w34) -> ()
  "error out" <- "error in (no error)"
